vi "test Writing To Empty String Handle.vi"(8 "error in (no error)":errorcluster, 11 "TestCase in":refnum<class "String Tests.lvclass">) -> (0 "error out":errorcluster, 3 "TestCase out":refnum<class "String Tests.lvclass">)   [LabVIEW 2020, in "String Tests.lvclass"]
uses:
  String Tests.lvclass
  <vilib>/Utility/file.llb/Application Directory.vi
  <vilib>/Utility/libraryn.llb/Check if File or Folder Exists.vi
  <vilib>/addons/_JKI Toolkits/VI Tester/TestCase.llb/TestCase.lvclass
  C:/Program Files/National Instruments/LabVIEW 2020/vi.lib/addons/_JKI Toolkits/VI Tester/TestCase.llb/TestCase.lvclass
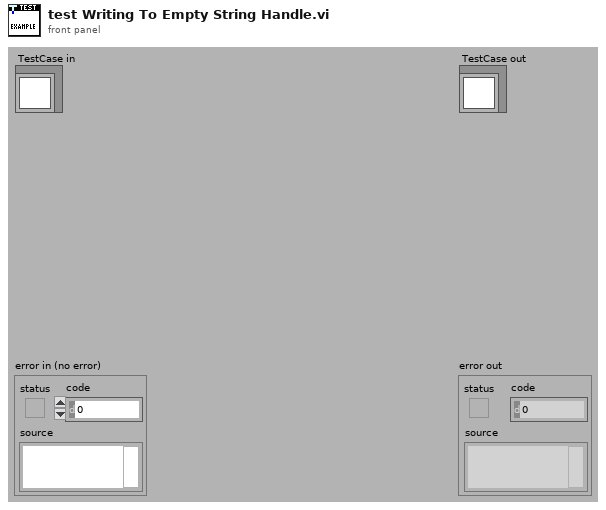
[diagram p1: front panel]
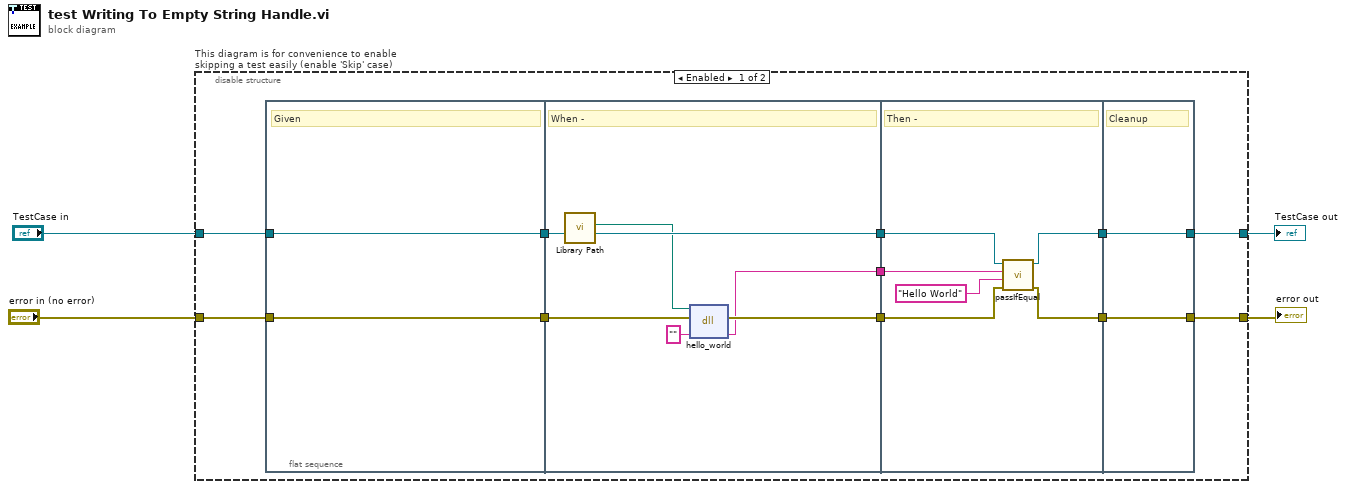
[diagram p0: block diagram]
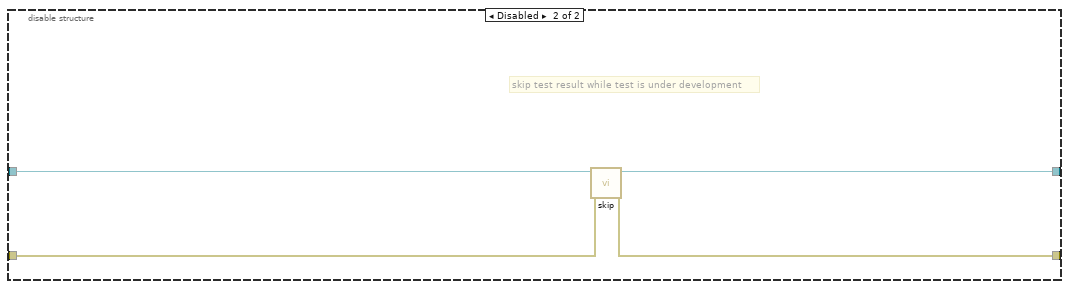
[diagram p2: hidden frame]
diagram:
  n1 = disable-structure "This diagram is for convenience to enable skipping a test easily (enable 'Skip' case)" shown="Enabled" {
    disable-tunnel: "TestCase in" -> [w9 w35]
    disable-tunnel: [w7 w33] -> w1
    disable-tunnel: [w6 w34] -> w3
    disable-tunnel: "error in (no error)" -> [w8 w32]
    frame Enabled {
      n2 = flat-sequence {
        tunnel: w8 -> [w16]
        tunnel: w9 -> [w17]
        tunnel: [w17] -> w15
        tunnel: [w16] -> w14
        tunnel: [w23] -> w13
        tunnel: [w21] -> w12
        tunnel: w15 -> [w23]
        tunnel: w14 -> [w20]
        tunnel: [w18] -> w5
        tunnel: [w28] -> w11
        tunnel: [w26] -> w10
        tunnel: w13 -> [w29]
        tunnel: w12 -> [w27]
        tunnel: w5 -> [w25]
        tunnel: [w30] -> w6
        tunnel: [w31] -> w7
        tunnel: w11 -> [w31]
        tunnel: w10 -> [w30]
        frame #0 {
          # "Given"
        }
        frame #1 {
          # "When -"
          n3 = call "Library Path.vi"() -> ("Library Path"=w22:path)  [unwired: 11 in]
          n4 = dll-call lib="C:/Users/JamesMcNally/Documents/RustInterop/Rust-LabVIEW-Interop/target/debug/labview_test_library.dll" fn="hello_world"(path in=w22, error in=w20, "string"="") -> (error out=w21:errorcluster, "string"=w18:string)  [unwired: 2 in, 1 out]
        }
        frame #2 {
          # "Then -"
          n5 = call-dynamic "passIfEqual.vi"("error in (no error)"=w27, "y"="Hello World" ("string"), "x"=w25, "TestCase in"=w29) -> ("error out"=w26:errorcluster, "TestCase out"=w28:refnum<class "String Tests.lvclass">)  [unwired: 6 in]
        }
        frame #3 {
          # "Cleanup"
        }
      }
    }
    frame Disabled {
      # "skip test result while test is under development"
      n6 = call <vilib>:"skip.vi"("error in (no error)"=w32, "TestCase in"=w35) -> ("error out"=w34:errorcluster, "TestCase out"=w33:refnum<class "String Tests.lvclass">)  [unwired: 8 in]
    }
  }
  "error out" <- w3
  "TestCase out" <- w1
